vi "ObtainQueue.vi"(8 "error in (no error)":errorcluster) -> (0 "error out":errorcluster, 3 "MessageQueue":refnum<queue>)   [LabVIEW 2014, in "AnalysisModule.lvlib"]
uses:
  AnalysisModule.lvlib
  PublicAPI/Arguments/Messages/clMessage.ctl
panel:
  # "This obtaind a queue and\nenqueues the \"Initialize\"\nMessage"
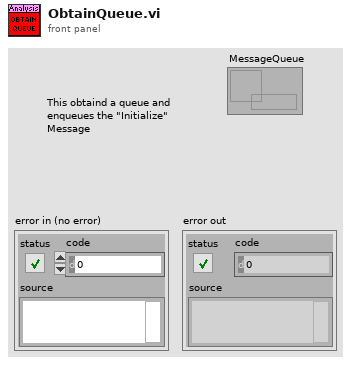
[diagram p1: front panel]
types:
  T1 = typedef "AnalysisModule.lvlib/clMessage.ctl" = cluster{"Message":string, "Message Data":variant}
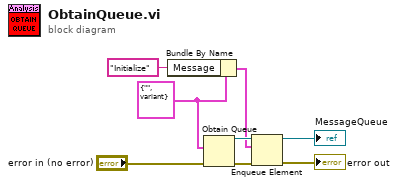
[diagram p0: block diagram]
diagram:
  w6 = T1 {"Message"="", "Message Data"=variant} ("clMessage")
  n1 = Bundle By Name(cluster=w6, "Message"="Initialize") -> (w4:T1)
  n2 = Obtain Queue(element data type=w6, error in (no error)="error in (no error)") -> (queue out=w7:refnum<queue>, error out=w3:errorcluster)  [unwired: 3 in, 1 out]
  n3 = Enqueue Element(queue=w7, element=w4, error in (no error)=w3) -> (queue out=→"MessageQueue":refnum<queue>, error out=→"error out":errorcluster)  [unwired: 1 in, 1 out]
